vi "Acquire Image from Camera.vi"(2 "Session In":T1, 3 "AutoBalance":bool, 4 "Set":bool, 5 "Stop (F)":bool, 7 "error in":errorcluster) -> (20 "Image Out":T2(plugin-control), 22 "Buffer Number Out":u32, 26 "Stopped":bool, 27 "error out":errorcluster)   [LabVIEW 2015]
doc: "Creates, and edits acquisitions using the NI Vision Acquisition Express VI.\n\nThe NI Vision Acquisition Wizard is launched by placing the Express VI on the block diagram. Select an acquisition source and configure an acquisition using NI-IMAQ, NI-IMAQdx, or simulate an acquisition by reading an AVI or image files from a folder. After an acquisition is configured, select controls and indicators to be able to programmatically set in LabVIEW. Double-click the Vision Acquisition Express VI to edit the acquisition.\n\nNote: Any images created by the Express VI need to be disposed after use. Use the IMAQ Dispose.vi to cleanup the images output by the Express VI when they are no longer needed."
uses:
  <vilib>/userdefined/High Color/IMAQdx.ctl
  <vilib>/vision/driver/IMAQdx.llb/IMAQdx Buffer Number Mode.ctl
  <vilib>/vision/driver/IMAQdx.llb/IMAQdx Acquisition Mode.ctl
  <vilib>/vision/driver/NI_Vision_Acquisition_Software.lvlib
  <resource>/objmgr/imaqdx.rc
panel:
  out "LostBufferCount":u32
  out "error out 2":errorcluster
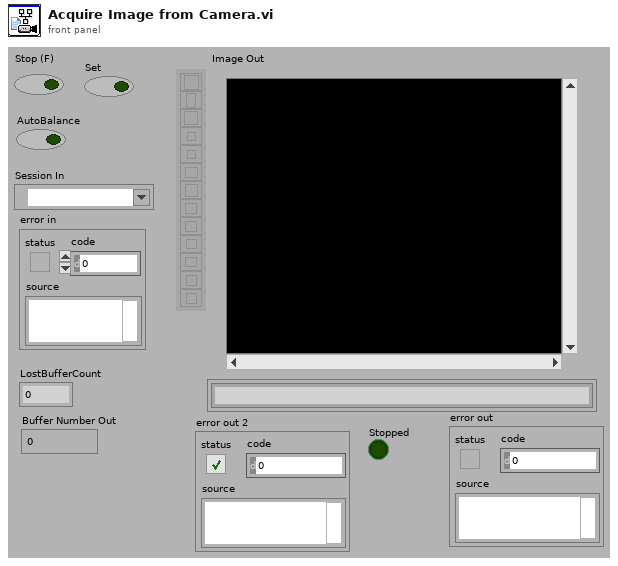
[diagram p1: front panel]
types:
  T1 = typedef "IMAQdx.ctl" = refnum<k21>
  T2 = typedef "IMAQ Image.ctl" = refnum<image>
  T3 = typedef "NI_Vision_Acquisition_Software.lvlib/IMAQdx Buffer Number Mode.ctl" = enum32{"Next", "Last", "Buffer Number", "Every", "Last New"}
  T4 = typedef "NI_Vision_Acquisition_Software.lvlib/IMAQdx Acquisition Mode.ctl" = enum32{"One Shot", "Continuous"}
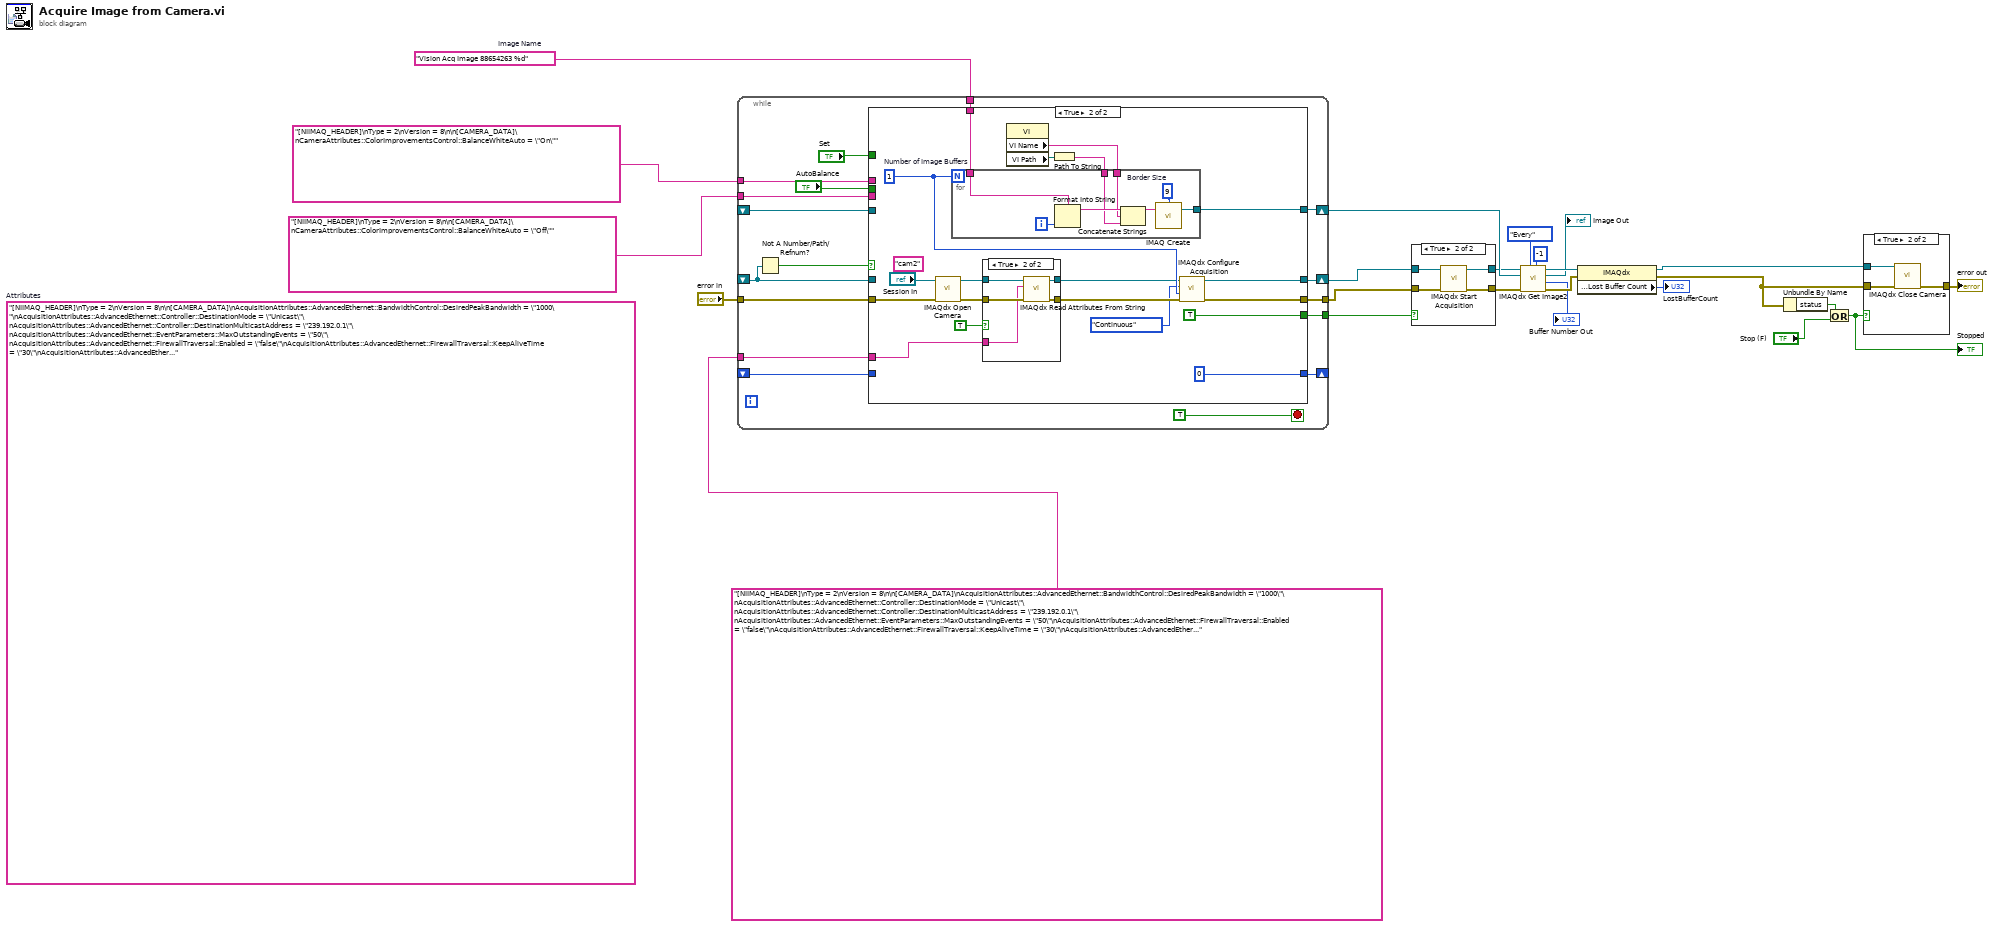
[diagram p0: block diagram]
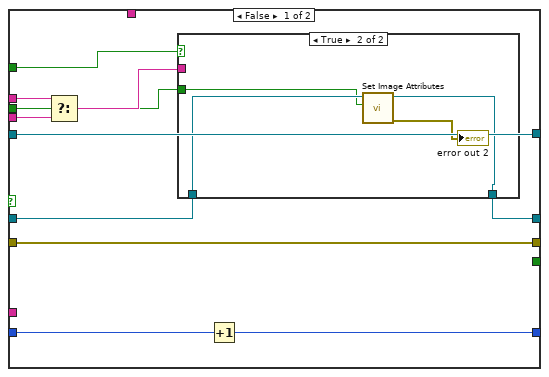
[diagram p4: hidden frame]
diagram:
  (unwired) "[NIIMAQ_HEADER]\nType = 2\nVersion = 8\n\n[CAMERA_DATA]\nAcquisitionAttributes::AdvancedEthernet::BandwidthControl::DesiredPeakBandwidth = \"1000\"\nAcquisitionAttributes::AdvancedEthernet::Controller::DestinationMode = \"Unicast\"\nAcquisitionAttributes::AdvancedEthernet::Controller::DestinationMulticastAddress = \"239.192.0.1\"\nAcquisitionAttributes::AdvancedEthernet::EventParameters::MaxOutstandingEvents = \"50\"\nAcquisitionAttributes::AdvancedEthernet::FirewallTraversal::Enabled = \"false\"\nAcquisitionAttributes::AdvancedEthernet::FirewallTraversal::KeepAliveTime = \"30\"\nAcquisitionAttributes::AdvancedEthernet::PacketReceptionParameters::KernelReceiveBufferSizeRequested = \"2000000\"\nAcquisitionAttributes::AdvancedEthernet::PacketReceptionParameters::MaximumPacketsPerReception = \"100\"\nAcquisitionAttributes::AdvancedEthernet::PacketReceptionParameters::PacketReceptionTimeout = \"450\"\nAcquisitionAttributes::AdvancedEthernet::PacketReceptionParameters::ThreadPriority = \"1\"\nAcquisitionAttributes::AdvancedEthernet::ResendParameters::MaxResendsPerPacket = \"25\"\nAcquisitionAttributes::AdvancedEthernet::ResendParameters::MemoryWindowSize = \"1024\"\nAcquisitionAttributes::AdvancedEthernet::ResendParameters::MissingPacketTimeout = \"2\"\nAcquisitionAttributes::AdvancedEthernet::ResendParameters::NewPacketTimeout = \"100\"\nAcquisitionAttributes::AdvancedEthernet::ResendParameters::ResendBatchingPercentage = \"10\"\nAcquisitionAttributes::AdvancedEthernet::ResendParameters::ResendResponseTimeout = \"2\"\nAcquisitionAttributes::AdvancedEthernet::ResendParameters::ResendsEnabled = \"true\"\nAcquisitionAttributes::AdvancedEthernet::ResendParameters::ResendThresholdPercentage = \"5\"\nAcquisitionAttributes::AdvancedEthernet::ResendParameters::ResendTimerResolution = \"1\"\nAcquisitionAttributes::AdvancedEthernet::TestPacketParameters::MaxTestPacketRetries = \"1\"\nAcquisitionAttributes::AdvancedEthernet::TestPacketParameters::TestPacketEnabled = \"true\"\nAcquisitionAttributes::AdvancedEthernet::TestPacketParameters::TestPacketTimeout = \"250\"\nAcquisitionAttributes::AdvancedGenicam::CommandTimeout = \"100\"\nAcquisitionAttributes::AdvancedGenicam::EventsEnabled = \"true\"\nAcquisitionAttributes::AdvancedGenicam::IgnoreCameraValidationErrors = \"false\"\nAcquisitionAttributes::Bayer::Algorithm = \"Bilinear\"\nAcquisitionAttributes::Bayer::GainB = \"1\"\nAcquisitionAttributes::Bayer::GainG = \"1\"\nAcquisitionAttributes::Bayer::GainR = \"1\"\nAcquisitionAttributes::Bayer::Pattern = \"Use hardware value\"\nAcquisitionAttributes::BitsPerPixel = \"Use hardware value\"\nAcquisitionAttributes::ChunkDataDecoding::ChunkDataDecodingEnabled = \"false\"\nAcquisitionAttributes::ChunkDataDecoding::MaximumChunkCopySize = \"64\"\nAcquisitionAttributes::IgnoreFirstFrame = \"false\"\nAcquisitionAttributes::ImageDecoderCopyMode = \"Auto\"\nAcquisitionAttributes::IncompleteBufferMode = \"Ignore\"\nAcquisitionAttributes::OutputImageType = \"Auto\"\nAcquisitionAttributes::OverwriteMode = \"Get Newest\"\nAcquisitionAttributes::PacketSize = \"8000\"\nAcquisitionAttributes::PixelSignedness = \"Use hardware value\"\nAcquisitionAttributes::ReceiveTimestampMode = \"None\"\nAcquisitionAttributes::ShiftPixelBits = \"false\"\nAcquisitionAttributes::SwapPixelBytes = \"false\"\nAcquisitionAttributes::Timeout = \"5000\"\nCameraAttributes::AcquisitionTrigger::AcquisitionFrameCount = \"1\"\nCameraAttributes::AcquisitionTrigger::AcquisitionFrameRateAbs = \"100\"\nCameraAttributes::AcquisitionTrigger::AcquisitionFrameRateEnable = \"true\"\nCameraAttributes::AcquisitionTrigger::ExposureAuto = \"On\"\nCameraAttributes::AcquisitionTrigger::ExposureMode = \"Timed\"\nCameraAttributes::AcquisitionTrigger::ExposureTimeRaw = \"1321\"\nCameraAttributes::AcquisitionTrigger::SensorReadoutMode = \"Normal\"\nCameraAttributes::AcquisitionTrigger::ShutterMode = \"Global\"\nCameraAttributes::AcquisitionTrigger::TriggerSelector = \"Acquisition Start\"\nCameraAttributes::AcquisitionTrigger::TriggerMode = \"Off\"\nCameraAttributes::AcquisitionTrigger::TriggerSource = \"Line 1\"\nCameraAttributes::AcquisitionTrigger::TriggerActivation = \"Rising Edge\"\nCameraAttributes::AcquisitionTrigger::TriggerDelayAbs = \"0\"\nCameraAttributes::AcquisitionTrigger::TriggerSelector = \"Frame Start\"\nCameraAttributes::AcquisitionTrigger::TriggerMode = \"Off\"\nCameraAttributes::AcquisitionTrigger::TriggerSource = \"Line 1\"\nCameraAttributes::AcquisitionTrigger::TriggerActivation = \"Rising Edge\"\nCameraAttributes::AcquisitionTrigger::TriggerDelayAbs = \"0\"\nCameraAttributes::AnalogControls::BlackLevelSelector = \"All\"\nCameraAttributes::AnalogControls::BlackLevelRaw = \"0\"\nCameraAttributes::AnalogControls::GainAuto = \"Off\"\nCameraAttributes::AnalogControls::GainSelector = \"All\"\nCameraAttributes::AnalogControls::GainRaw = \"136\"\nCameraAttributes::AnalogControls::GammaEnable = \"true\"\nCameraAttributes::AnalogControls::GammaSelector = \"SRGB\"\nCameraAttributes::AOI::CenterX = \"false\"\nCameraAttributes::AOI::CenterY = \"false\"\nCameraAttributes::AOI::Height = \"600\"\nCameraAttributes::AOI::OffsetX = \"16\"\nCameraAttributes::AOI::OffsetY = \"16\"\nCameraAttributes::AOI::Width = \"800\"\nCameraAttributes::AutoFunctions::AutoExposureTimeAbsLowerLimit = \"112\"\nCameraAttributes::AutoFunctions::AutoExposureTimeAbsUpperLimit = \"500000\"\nCameraAttributes::AutoFunctions::AutoFunctionAOIs::AutoFunctionAOISelector = \"AOI 1\"\nCameraAttributes::AutoFunctions::AutoFunctionAOIs::AutoFunctionAOIWidth = \"800\"\nCameraAttributes::AutoFunctions::AutoFunctionAOIs::AutoFunctionAOIHeight = \"600\"\nCameraAttributes::AutoFunctions::AutoFunctionAOIs::AutoFunctionAOIOffsetX = \"16\"\nCameraAttributes::AutoFunctions::AutoFunctionAOIs::AutoFunctionAOIOffsetY = \"16\"\nCameraAttributes::AutoFunctions::AutoFunctionAOIs::AutoFunctionAOISelector = \"AOI 2\"\nCameraAttributes::AutoFunctions::AutoFunctionAOIs::AutoFunctionAOIWidth = \"800\"\nCameraAttributes::AutoFunctions::AutoFunctionAOIs::AutoFunctionAOIHeight = \"600\"\nCameraAttributes::AutoFunctions::AutoFunctionAOIs::AutoFunctionAOIOffsetX = \"16\"\nCameraAttributes::AutoFunctions::AutoFunctionAOIs::AutoFunctionAOIOffsetY = \"16\"\nCameraAttributes::AutoFunctions::AutoFunctionProfile = \"Gain at minimum\"\nCameraAttributes::AutoFunctions::AutoGainRawLowerLimit = \"136\"\nCameraAttributes::AutoFunctions::AutoGainRawUpperLimit = \"542\"\nCameraAttributes::AutoFunctions::AutoTargetValue = \"128\"\nCameraAttributes::AutoFunctions::BalanceWhiteAdjustmentDampingRaw = \"1000\"\nCameraAttributes::AutoFunctions::GrayValueAdjustmentDampingRaw = \"700\"\nCameraAttributes::ChunkDataStreams::ChunkModeActive = \"false\"\nCameraAttributes::ColorImprovementsControl::BalanceRatioSelector = \"Red\"\nCameraAttributes::ColorImprovementsControl::BalanceRatioRaw = \"73\"\nCameraAttributes::ColorImprovementsControl::BalanceRatioSelector = \"Green\"\nCameraAttributes::ColorImprovementsControl::BalanceRatioRaw = \"64\"\nCameraAttributes::ColorImprovementsControl::BalanceRatioSelector = \"Blue\"\nCameraAttributes::ColorImprovementsControl::BalanceRatioRaw = \"101\"\nCameraAttributes::ColorImprovementsControl::BalanceRatioSelector = \"Red\"\nCameraAttributes::ColorImprovementsControl::BalanceWhiteAuto = \"On\"\nCameraAttributes::ColorImprovementsControl::ColorAdjustmentEnable = \"true\"\nCameraAttributes::ColorImprovementsControl::ColorAdjustmentSelector = \"Red\"\nCameraAttributes::ColorImprovementsControl::ColorAdjustmentHueRaw = \"-3\"\nCameraAttributes::ColorImprovementsControl::ColorAdjustmentSaturationRaw = \"128\"\nCameraAttributes::ColorImprovementsControl::ColorAdjustmentSelector = \"Yellow\"\nCameraAttributes::ColorImprovementsControl::ColorAdjustmentHueRaw = \"7\"\nCameraAttributes::ColorImprovementsControl::ColorAdjustmentSaturationRaw = \"124\"\nCameraAttributes::ColorImprovementsControl::ColorAdjustmentSelector = \"Green\"\nCameraAttributes::ColorImprovementsControl::ColorAdjustmentHueRaw = \"0\"\nCameraAttributes::ColorImprovementsControl::ColorAdjustmentSaturationRaw = \"138\"\nCameraAttributes::ColorImprovementsControl::ColorAdjustmentSelector = \"Cyan\"\nCameraAttributes::ColorImprovementsControl::ColorAdjustmentHueRaw = \"9\"\nCameraAttributes::ColorImprovementsControl::ColorAdjustmentSaturationRaw = \"135\"\nCameraAttributes::ColorImprovementsControl::ColorAdjustmentSelector = \"Blue\"\nCameraAttributes::ColorImprovementsControl::ColorAdjustmentHueRaw = \"-5\"\nCameraAttributes::ColorImprovementsControl::ColorAdjustmentSaturationRaw = \"126\"\nCameraAttributes::ColorImprovementsControl::ColorAdjustmentSelector = \"Magenta\"\nCameraAttributes::ColorImprovementsControl::ColorAdjustmentHueRaw = \"25\"\nCameraAttributes::ColorImprovementsControl::ColorAdjustmentSaturationRaw = \"134\"\nCameraAttributes::ColorImprovementsControl::ColorAdjustmentSelector = \"Red\"\nCameraAttributes::ColorImprovementsControl::ColorTransformationMatrixFactorRaw = \"65536\"\nCameraAttributes::ColorImprovementsControl::ColorTransformationSelector = \"RGB to RGB\"\nCameraAttributes::ColorImprovementsControl::LightSourceSelector = \"Daylight 5000 Kelvin\"\nCameraAttributes::DigitalIO::LineSelector = \"Line 1\"\nCameraAttributes::DigitalIO::LineMode = \"Input\"\nCameraAttributes::DigitalIO::LineDebouncerTimeRaw = \"10000\"\nCameraAttributes::DigitalIO::LineInverter = \"false\"\nCameraAttributes::DigitalIO::LineFormat = \"Opto-coupled\"\nCameraAttributes::DigitalIO::LineSelector = \"Line 2\"\nCameraAttributes::DigitalIO::LineMode = \"Output\"\nCameraAttributes::DigitalIO::LineInverter = \"false\"\nCameraAttributes::DigitalIO::LineSource = \"User Output 1\"\nCameraAttributes::DigitalIO::LineFormat = \"Opto-coupled\"\nCameraAttributes::DigitalIO::MinOutPulseWidthRaw = \"0\"\nCameraAttributes::DigitalIO::LineSelector = \"Line 3\"\nCameraAttributes::DigitalIO::LineMode = \"Input\"\nCameraAttributes::DigitalIO::LineDebouncerTimeRaw = \"0\"\nCameraAttributes::DigitalIO::LineInverter = \"false\"\nCameraAttributes::DigitalIO::LineFormat = \"TTL\"\nCameraAttributes::DigitalIO::LineSelector = \"Line 1\"\nCameraAttributes::DigitalIO::SyncUserOutputValueAll = \"0\"\nCameraAttributes::DigitalIO::UserOutputValueAll = \"0\"\nCameraAttributes::EventsGeneration::EventSelector = \"Exposure End\"\nCameraAttributes::EventsGeneration::EventNotification = \"Notification Off\"\nCameraAttributes::EventsGeneration::EventSelector = \"Frame Start Overtrigger\"\nCameraAttributes::EventsGeneration::EventNotification = \"Notification Off\"\nCameraAttributes::EventsGeneration::EventSelector = \"Acquisition Start Overtrigger\"\nCameraAttributes::EventsGeneration::EventNotification = \"Notification Off\"\nCameraAttributes::EventsGeneration::EventSelector = \"Frame Start\"\nCameraAttributes::EventsGeneration::EventNotification = \"Notification Off\"\nCameraAttributes::EventsGeneration::EventSelector = \"Acquisition Start\"\nCameraAttributes::EventsGeneration::EventNotification = \"Notification Off\"\nCameraAttributes::EventsGeneration::EventSelector = \"Critical Temperature\"\nCameraAttributes::EventsGeneration::EventNotification = \"Notification Off\"\nCameraAttributes::EventsGeneration::EventSelector = \"Over Temperature\"\nCameraAttributes::EventsGeneration::EventNotification = \"Notification Off\"\nCameraAttributes::EventsGeneration::EventSelector = \"Action Late\"\nCameraAttributes::EventsGeneration::EventNotification = \"Notification Off\"\nCameraAttributes::EventsGeneration::EventSelector = \"Frame Start Wait\"\nCameraAttributes::EventsGeneration::EventNotification = \"Notification Off\"\nCameraAttributes::EventsGeneration::EventSelector = \"Acquisition Start Wait\"\nCameraAttributes::EventsGeneration::EventNotification = \"Notification Off\"\nCameraAttributes::EventsGeneration::EventSelector = \"Event Overrun\"\nCameraAttributes::EventsGeneration::EventNotification = \"Notification Off\"\nCameraAttributes::EventsGeneration::EventSelector = \"Exposure End\"\nCameraAttributes::ExpertFeatureAccess::ExpertFeatureAccessSelector = \"Expert Feature 1\"\nCameraAttributes::ExpertFeatureAccess::ExpertFeatureAccessSelector = \"Expert Feature 2\"\nCameraAttributes::ExpertFeatureAccess::ExpertFeatureAccessSelector = \"Expert Feature 3\"\nCameraAttributes::ExpertFeatureAccess::ExpertFeatureAccessSelector = \"Expert Feature 4\"\nCameraAttributes::ExpertFeatureAccess::ExpertFeatureAccessSelector = \"Expert Feature 5\"\nCameraAttributes::ExpertFeatureAccess::ExpertFeatureAccessSelector = \"Expert Feature 6\"\nCameraAttributes::ExpertFeatureAccess::ExpertFeatureAccessSelector = \"Expert Feature 7\"\nCameraAttributes::ExpertFeatureAccess::ExpertFeatureAccessSelector = \"Expert Feature 8\"\nCameraAttributes::ExpertFeatureAccess::ExpertFeatureAccessSelector = \"Expert Feature 9\"\nCameraAttributes::ExpertFeatureAccess::ExpertFeatureAccessSelector = \"Expert Feature 1\"\nCameraAttributes::ImageFormat::PixelFormat = \"Bayer BG 8\"\nCameraAttributes::ImageFormat::ReverseX = \"false\"\nCameraAttributes::ImageFormat::ReverseY = \"false\"\nCameraAttributes::ImageFormat::TestImageSelector = \"Test Image Off\"\nCameraAttributes::LUTControls::LUTSelector = \"Luminance LUT\"\nCameraAttributes::LUTControls::LUTEnable = \"false\"\nCameraAttributes::LUTControls::LUTValueAll = \"000000000000000000000002000000000000000400000000000000060000000000000008000000000000000A000000000000000C000000000000000E00000000000000100000000000000012000000000000001400000000000000160000000000000018000000000000001A000000000000001C000000000000001E00000000000000200000000000000022000000000000002400000000000000260000000000000028000000000000002A000000000000002C000000000000002E00000000000000300000000000000032000000000000003400000000000000360000000000000038000000000000003A000000000000003C000000000000003E00000000000000400000000000000042000000000000004400000000000000460000000000000048000000000000004A000000000000004C000000000000004E00000000000000500000000000000052000000000000005400000000000000560000000000000058000000000000005A000000000000005C000000000000005E00000000000000600000000000000062000000000000006400000000000000660000000000000068000000000000006A000000000000006C000000000000006E00000000000000700000000000000072000000000000007400000000000000760000000000000078000000000000007A000000000000007C000000000000007E00000000000000800000000000000082000000000000008400000000000000860000000000000088000000000000008A000000000000008C000000000000008E00000000000000900000000000000092000000000000009400000000000000960000000000000098000000000000009A000000000000009C000000000000009E00000000000000A000000000000000A200000000000000A400000000000000A600000000000000A800000000000000AA00000000000000AC00000000000000AE00000000000000B000000000000000B200000000000000B400000000000000B600000000000000B800000000000000BA00000000000000BC00000000000000BE00000000000000C000000000000000C200000000000000C400000000000000C600000000000000C800000000000000CA00000000000000CC00000000000000CE00000000000000D000000000000000D200000000000000D400000000000000D600000000000000D800000000000000DA00000000000000DC00000000000000DE00000000000000E000000000000000E200000000000000E400000000000000E600000000000000E800000000000000EA00000000000000EC00000000000000EE00000000000000F000000000000000F200000000000000F400000000000000F600000000000000F800000000000000FA00000000000000FC00000000000000FE00000000000001000000000000000102000000000000010400000000000001060000000000000108000000000000010A000000000000010C000000000000010E00000000000001100000000000000112000000000000011400000000000001160000000000000118000000000000011A000000000000011C000000000000011E00000000000001200000000000000122000000000000012400000000000001260000000000000128000000000000012A000000000000012C000000000000012E00000000000001300000000000000132000000000000013400000000000001360000000000000138000000000000013A000000000000013C000000000000013E00000000000001400000000000000142000000000000014400000000000001460000000000000148000000000000014A000000000000014C000000000000014E00000000000001500000000000000152000000000000015400000000000001560000000000000158000000000000015A000000000000015C000000000000015E00000000000001600000000000000162000000000000016400000000000001660000000000000168000000000000016A000000000000016C000000000000016E00000000000001700000000000000172000000000000017400000000000001760000000000000178000000000000017A000000000000017C000000000000017E00000000000001800000000000000182000000000000018400000000000001860000000000000188000000000000018A000000000000018C000000000000018E00000000000001900000000000000192000000000000019400000000000001960000000000000198000000000000019A000000000000019C000000000000019E00000000000001A000000000000001A200000000000001A400000000000001A600000000000001A800000000000001AA00000000000001AC00000000000001AE00000000000001B000000000000001B200000000000001B400000000000001B600000000000001B800000000000001BA00000000000001BC00000000000001BE00000000000001C000000000000001C200000000000001C400000000000001C600000000000001C800000000000001CA00000000000001CC00000000000001CE00000000000001D000000000000001D200000000000001D400000000000001D600000000000001D800000000000001DA00000000000001DC00000000000001DE00000000000001E000000000000001E200000000000001E400000000000001E600000000000001E800000000000001EA00000000000001EC00000000000001EE00000000000001F000000000000001F200000000000001F400000000000001F600000000000001F800000000000001FA00000000000001FC00000000000001FE00000000000002000000000000000202000000000000020400000000000002060000000000000208000000000000020A000000000000020C000000000000020E00000000000002100000000000000212000000000000021400000000000002160000000000000218000000000000021A000000000000021C000000000000021E00000000000002200000000000000222000000000000022400000000000002260000000000000228000000000000022A000000000000022C000000000000022E00000000000002300000000000000232000000000000023400000000000002360000000000000238000000000000023A000000000000023C000000000000023E00000000000002400000000000000242000000000000024400000000000002460000000000000248000000000000024A000000000000024C000000000000024E00000000000002500000000000000252000000000000025400000000000002560000000000000258000000000000025A000000000000025C000000000000025E00000000000002600000000000000262000000000000026400000000000002660000000000000268000000000000026A000000000000026C000000000000026E00000000000002700000000000000272000000000000027400000000000002760000000000000278000000000000027A000000000000027C000000000000027E00000000000002800000000000000282000000000000028400000000000002860000000000000288000000000000028A000000000000028C000000000000028E00000000000002900000000000000292000000000000029400000000000002960000000000000298000000000000029A000000000000029C000000000000029E00000000000002A000000000000002A200000000000002A400000000000002A600000000000002A800000000000002AA00000000000002AC00000000000002AE00000000000002B000000000000002B200000000000002B400000000000002B600000000000002B800000000000002BA00000000000002BC00000000000002BE00000000000002C000000000000002C200000000000002C400000000000002C600000000000002C800000000000002CA00000000000002CC00000000000002CE00000000000002D000000000000002D200000000000002D400000000000002D600000000000002D800000000000002DA00000000000002DC00000000000002DE00000000000002E000000000000002E200000000000002E400000000000002E600000000000002E800000000000002EA00000000000002EC00000000000002EE00000000000002F000000000000002F200000000000002F400000000000002F600000000000002F800000000000002FA00000000000002FC00000000000002FE00000000000003000000000000000302000000000000030400000000000003060000000000000308000000000000030A000000000000030C000000000000030E00000000000003100000000000000312000000000000031400000000000003160000000000000318000000000000031A000000000000031C000000000000031E00000000000003200000000000000322000000000000032400000000000003260000000000000328000000000000032A000000000000032C000000000000032E00000000000003300000000000000332000000000000033400000000000003360000000000000338000000000000033A000000000000033C000000000000033E00000000000003400000000000000342000000000000034400000000000003460000000000000348000000000000034A000000000000034C000000000000034E00000000000003500000000000000352000000000000035400000000000003560000000000000358000000000000035A000000000000035C000000000000035E00000000000003600000000000000362000000000000036400000000000003660000000000000368000000000000036A000000000000036C000000000000036E00000000000003700000000000000372000000000000037400000000000003760000000000000378000000000000037A000000000000037C000000000000037E00000000000003800000000000000382000000000000038400000000000003860000000000000388000000000000038A000000000000038C000000000000038E00000000000003900000000000000392000000000000039400000000000003960000000000000398000000000000039A000000000000039C000000000000039E00000000000003A000000000000003A200000000000003A400000000000003A600000000000003A800000000000003AA00000000000003AC00000000000003AE00000000000003B000000000000003B200000000000003B400000000000003B600000000000003B800000000000003BA00000000000003BC00000000000003BE00000000000003C000000000000003C200000000000003C400000000000003C600000000000003C800000000000003CA00000000000003CC00000000000003CE00000000000003D000000000000003D200000000000003D400000000000003D600000000000003D800000000000003DA00000000000003DC00000000000003DE00000000000003E000000000000003E200000000000003E400000000000003E600000000000003E800000000000003EA00000000000003EC00000000000003EE00000000000003F000000000000003F200000000000003F400000000000003F600000000000003F800000000000003FA00000000000003FC00000000000003FE00000000\"\nCameraAttributes::RemoveParamLimits::ParameterSelector = \"Gain\"\nCameraAttributes::RemoveParamLimits::RemoveLimits = \"false\"\nCameraAttributes::RemoveParamLimits::ParameterSelector = \"Exposure Time\"\nCameraAttributes::RemoveParamLimits::RemoveLimits = \"false\"\nCameraAttributes::RemoveParamLimits::ParameterSelector = \"Target Gray Value\"\nCameraAttributes::RemoveParamLimits::RemoveLimits = \"false\"\nCameraAttributes::RemoveParamLimits::ParameterSelector = \"Gain\"\nCameraAttributes::TimerControls::CounterSelector = \"Counter 1\"\nCameraAttributes::TimerControls::CounterEventSource = \"Frame Trigger\"\nCameraAttributes::TimerControls::CounterResetSource = \"Off\"\nCameraAttributes::TimerControls::CounterSelector = \"Counter 2\"\nCameraAttributes::TimerControls::CounterEventSource = \"Frame Start\"\nCameraAttributes::TimerControls::CounterResetSource = \"Off\"\nCameraAttributes::TimerControls::TimerDelayTimebaseAbs = \"1\"\nCameraAttributes::TimerControls::TimerDurationTimebaseAbs = \"1\"\nCameraAttributes::TimerControls::TimerSelector = \"Timer 1\"\nCameraAttributes::TimerControls::TimerDurationAbs = \"4095\"\nCameraAttributes::TimerControls::TimerDurationRaw = \"4095\"\nCameraAttributes::TimerControls::TimerDelayAbs = \"0\"\nCameraAttributes::TimerControls::TimerDelayRaw = \"0\"\nCameraAttributes::TransportLayer::GevStreamChannelSelector = \"Stream Channel 0\"\nCameraAttributes::TransportLayer::GevSCFTD = \"0\"\nCameraAttributes::TransportLayer::GevSCBWR = \"10\"\nCameraAttributes::TransportLayer::GevSCBWRA = \"10\"\nCameraAttributes::UserDefinedValues::UserDefinedValueSelector = \"Value 1\"\nCameraAttributes::UserDefinedValues::UserDefinedValue = \"0\"\nCameraAttributes::UserDefinedValues::UserDefinedValueSelector = \"Value 2\"\nCameraAttributes::UserDefinedValues::UserDefinedValue = \"0\"\nCameraAttributes::UserDefinedValues::UserDefinedValueSelector = \"Value 3\"\nCameraAttributes::UserDefinedValues::UserDefinedValue = \"0\"\nCameraAttributes::UserDefinedValues::UserDefinedValueSelector = \"Value 4\"\nCameraAttributes::UserDefinedValues::UserDefinedValue = \"0\"\nCameraAttributes::UserDefinedValues::UserDefinedValueSelector = \"Value 5\"\nCameraAttributes::UserDefinedValues::UserDefinedValue = \"0\"\nCameraAttributes::UserDefinedValues::UserDefinedValueSelector = \"Value 1\"\n"  # Attributes
  w6 = "Vision Acq Image 88654263 %d"  # Image Name
  n1 = while {
    shift-right: [w41] -> w17
    shift-left: _ -> [w33]
    tunnel: [w40] -> w23
    tunnel: "error in" -> [w39]
    shift-right: [w37] -> w19
    shift-left: _ -> [w36]
    shift-right: [w35] -> _
    shift-left: _ -> [w34]
    tunnel: [w32] -> w14
    tunnel: w6 -> [w31]
    tunnel: "[NIIMAQ_HEADER]\nType = 2\nVersion = 8\n\n[CAMERA_DATA]\nAcquisitionAttributes::AdvancedEthernet::BandwidthControl::DesiredPeakBandwidth = \"1000\"\nAcquisitionAttributes::AdvancedEthernet::Controller::DestinationMode = \"Unicast\"\nAcquisitionAttributes::AdvancedEthernet::Controller::DestinationMulticastAddress = \"239.192.0.1\"\nAcquisitionAttributes::AdvancedEthernet::EventParameters::MaxOutstandingEvents = \"50\"\nAcquisitionAttributes::AdvancedEthernet::FirewallTraversal::Enabled = \"false\"\nAcquisitionAttributes::AdvancedEthernet::FirewallTraversal::KeepAliveTime = \"30\"\nAcquisitionAttributes::AdvancedEthernet::PacketReceptionParameters::KernelReceiveBufferSizeRequested = \"2000000\"\nAcquisitionAttributes::AdvancedEthernet::PacketReceptionParameters::MaximumPacketsPerReception = \"100\"\nAcquisitionAttributes::AdvancedEthernet::PacketReceptionParameters::PacketReceptionTimeout = \"450\"\nAcquisitionAttributes::AdvancedEthernet::PacketReceptionParameters::ThreadPriority = \"1\"\nAcquisitionAttributes::AdvancedEthernet::ResendParameters::MaxResendsPerPacket = \"25\"\nAcquisitionAttributes::AdvancedEthernet::ResendParameters::MemoryWindowSize = \"1024\"\nAcquisitionAttributes::AdvancedEthernet::ResendParameters::MissingPacketTimeout = \"2\"\nAcquisitionAttributes::AdvancedEthernet::ResendParameters::NewPacketTimeout = \"100\"\nAcquisitionAttributes::AdvancedEthernet::ResendParameters::ResendBatchingPercentage = \"10\"\nAcquisitionAttributes::AdvancedEthernet::ResendParameters::ResendResponseTimeout = \"2\"\nAcquisitionAttributes::AdvancedEthernet::ResendParameters::ResendsEnabled = \"true\"\nAcquisitionAttributes::AdvancedEthernet::ResendParameters::ResendThresholdPercentage = \"5\"\nAcquisitionAttributes::AdvancedEthernet::ResendParameters::ResendTimerResolution = \"1\"\nAcquisitionAttributes::AdvancedEthernet::TestPacketParameters::MaxTestPacketRetries = \"1\"\nAcquisitionAttributes::AdvancedEthernet::TestPacketParameters::TestPacketEnabled = \"true\"\nAcquisitionAttributes::AdvancedEthernet::TestPacketParameters::TestPacketTimeout = \"250\"\nAcquisitionAttributes::AdvancedGenicam::CommandTimeout = \"100\"\nAcquisitionAttributes::AdvancedGenicam::EventsEnabled = \"true\"\nAcquisitionAttributes::AdvancedGenicam::IgnoreCameraValidationErrors = \"false\"\nAcquisitionAttributes::Bayer::Algorithm = \"Bilinear\"\nAcquisitionAttributes::Bayer::GainB = \"0.877538834319664396\"\nAcquisitionAttributes::Bayer::GainG = \"0.864790174043026272\"\nAcquisitionAttributes::Bayer::GainR = \"0.854384386209105284\"\nAcquisitionAttributes::Bayer::Pattern = \"Use hardware value\"\nAcquisitionAttributes::BitsPerPixel = \"Use hardware value\"\nAcquisitionAttributes::ChunkDataDecoding::ChunkDataDecodingEnabled = \"false\"\nAcquisitionAttributes::ChunkDataDecoding::MaximumChunkCopySize = \"64\"\nAcquisitionAttributes::IgnoreFirstFrame = \"false\"\nAcquisitionAttributes::ImageDecoderCopyMode = \"Auto\"\nAcquisitionAttributes::IncompleteBufferMode = \"Ignore\"\nAcquisitionAttributes::OutputImageType = \"Auto\"\nAcquisitionAttributes::OverwriteMode = \"Get Newest\"\nAcquisitionAttributes::PacketSize = \"8000\"\nAcquisitionAttributes::PixelSignedness = \"Use hardware value\"\nAcquisitionAttributes::ReceiveTimestampMode = \"None\"\nAcquisitionAttributes::ShiftPixelBits = \"false\"\nAcquisitionAttributes::SwapPixelBytes = \"false\"\nAcquisitionAttributes::Timeout = \"5000\"\nCameraAttributes::AcquisitionTrigger::AcquisitionFrameCount = \"1\"\nCameraAttributes::AcquisitionTrigger::AcquisitionFrameRateAbs = \"100\"\nCameraAttributes::AcquisitionTrigger::AcquisitionFrameRateEnable = \"true\"\nCameraAttributes::AcquisitionTrigger::ExposureAuto = \"Off\"\nCameraAttributes::AcquisitionTrigger::ExposureMode = \"Timed\"\nCameraAttributes::AcquisitionTrigger::ExposureTimeRaw = \"2500\"\nCameraAttributes::AcquisitionTrigger::SensorReadoutMode = \"Normal\"\nCameraAttributes::AcquisitionTrigger::ShutterMode = \"Global\"\nCameraAttributes::AcquisitionTrigger::TriggerSelector = \"Acquisition Start\"\nCameraAttributes::AcquisitionTrigger::TriggerMode = \"Off\"\nCameraAttributes::AcquisitionTrigger::TriggerSource = \"Line 1\"\nCameraAttributes::AcquisitionTrigger::TriggerActivation = \"Rising Edge\"\nCameraAttributes::AcquisitionTrigger::TriggerDelayAbs = \"0\"\nCameraAttributes::AcquisitionTrigger::TriggerSelector = \"Frame Start\"\nCameraAttributes::AcquisitionTrigger::TriggerMode = \"Off\"\nCameraAttributes::AcquisitionTrigger::TriggerSource = \"Line 1\"\nCameraAttributes::AcquisitionTrigger::TriggerActivation = \"Rising Edge\"\nCameraAttributes::AcquisitionTrigger::TriggerDelayAbs = \"0\"\nCameraAttributes::AnalogControls::BlackLevelSelector = \"All\"\nCameraAttributes::AnalogControls::BlackLevelRaw = \"0\"\nCameraAttributes::AnalogControls::GainAuto = \"Off\"\nCameraAttributes::AnalogControls::GainSelector = \"All\"\nCameraAttributes::AnalogControls::GainRaw = \"136\"\nCameraAttributes::AnalogControls::GammaEnable = \"true\"\nCameraAttributes::AnalogControls::GammaSelector = \"SRGB\"\nCameraAttributes::AOI::CenterX = \"false\"\nCameraAttributes::AOI::CenterY = \"false\"\nCameraAttributes::AOI::Height = \"600\"\nCameraAttributes::AOI::OffsetX = \"0\"\nCameraAttributes::AOI::OffsetY = \"0\"\nCameraAttributes::AOI::Width = \"800\"\nCameraAttributes::AutoFunctions::AutoExposureTimeAbsLowerLimit = \"112\"\nCameraAttributes::AutoFunctions::AutoExposureTimeAbsUpperLimit = \"500000\"\nCameraAttributes::AutoFunctions::AutoFunctionAOIs::AutoFunctionAOISelector = \"AOI 1\"\nCameraAttributes::AutoFunctions::AutoFunctionAOIs::AutoFunctionAOIWidth = \"800\"\nCameraAttributes::AutoFunctions::AutoFunctionAOIs::AutoFunctionAOIHeight = \"600\"\nCameraAttributes::AutoFunctions::AutoFunctionAOIs::AutoFunctionAOIOffsetX = \"16\"\nCameraAttributes::AutoFunctions::AutoFunctionAOIs::AutoFunctionAOIOffsetY = \"16\"\nCameraAttributes::AutoFunctions::AutoFunctionAOIs::AutoFunctionAOISelector = \"AOI 2\"\nCameraAttributes::AutoFunctions::AutoFunctionAOIs::AutoFunctionAOIWidth = \"800\"\nCameraAttributes::AutoFunctions::AutoFunctionAOIs::AutoFunctionAOIHeight = \"600\"\nCameraAttributes::AutoFunctions::AutoFunctionAOIs::AutoFunctionAOIOffsetX = \"16\"\nCameraAttributes::AutoFunctions::AutoFunctionAOIs::AutoFunctionAOIOffsetY = \"16\"\nCameraAttributes::AutoFunctions::AutoFunctionProfile = \"Gain at minimum\"\nCameraAttributes::AutoFunctions::AutoGainRawLowerLimit = \"136\"\nCameraAttributes::AutoFunctions::AutoGainRawUpperLimit = \"542\"\nCameraAttributes::AutoFunctions::AutoTargetValue = \"128\"\nCameraAttributes::AutoFunctions::BalanceWhiteAdjustmentDampingRaw = \"1000\"\nCameraAttributes::AutoFunctions::GrayValueAdjustmentDampingRaw = \"700\"\nCameraAttributes::ChunkDataStreams::ChunkModeActive = \"false\"\nCameraAttributes::ColorImprovementsControl::BalanceRatioSelector = \"Red\"\nCameraAttributes::ColorImprovementsControl::BalanceRatioRaw = \"158\"\nCameraAttributes::ColorImprovementsControl::BalanceRatioSelector = \"Green\"\nCameraAttributes::ColorImprovementsControl::BalanceRatioRaw = \"117\"\nCameraAttributes::ColorImprovementsControl::BalanceRatioSelector = \"Blue\"\nCameraAttributes::ColorImprovementsControl::BalanceRatioRaw = \"64\"\nCameraAttributes::ColorImprovementsControl::BalanceRatioSelector = \"Red\"\nCameraAttributes::ColorImprovementsControl::BalanceWhiteAuto = \"Off\"\nCameraAttributes::ColorImprovementsControl::ColorAdjustmentEnable = \"true\"\nCameraAttributes::ColorImprovementsControl::ColorAdjustmentSelector = \"Red\"\nCameraAttributes::ColorImprovementsControl::ColorAdjustmentHueRaw = \"-3\"\nCameraAttributes::ColorImprovementsControl::ColorAdjustmentSaturationRaw = \"128\"\nCameraAttributes::ColorImprovementsControl::ColorAdjustmentSelector = \"Yellow\"\nCameraAttributes::ColorImprovementsControl::ColorAdjustmentHueRaw = \"7\"\nCameraAttributes::ColorImprovementsControl::ColorAdjustmentSaturationRaw = \"124\"\nCameraAttributes::ColorImprovementsControl::ColorAdjustmentSelector = \"Green\"\nCameraAttributes::ColorImprovementsControl::ColorAdjustmentHueRaw = \"0\"\nCameraAttributes::ColorImprovementsControl::ColorAdjustmentSaturationRaw = \"138\"\nCameraAttributes::ColorImprovementsControl::ColorAdjustmentSelector = \"Cyan\"\nCameraAttributes::ColorImprovementsControl::ColorAdjustmentHueRaw = \"9\"\nCameraAttributes::ColorImprovementsControl::ColorAdjustmentSaturationRaw = \"135\"\nCameraAttributes::ColorImprovementsControl::ColorAdjustmentSelector = \"Blue\"\nCameraAttributes::ColorImprovementsControl::ColorAdjustmentHueRaw = \"-5\"\nCameraAttributes::ColorImprovementsControl::ColorAdjustmentSaturationRaw = \"126\"\nCameraAttributes::ColorImprovementsControl::ColorAdjustmentSelector = \"Magenta\"\nCameraAttributes::ColorImprovementsControl::ColorAdjustmentHueRaw = \"25\"\nCameraAttributes::ColorImprovementsControl::ColorAdjustmentSaturationRaw = \"134\"\nCameraAttributes::ColorImprovementsControl::ColorAdjustmentSelector = \"Red\"\nCameraAttributes::ColorImprovementsControl::ColorTransformationMatrixFactorRaw = \"65536\"\nCameraAttributes::ColorImprovementsControl::ColorTransformationSelector = \"RGB to RGB\"\nCameraAttributes::ColorImprovementsControl::LightSourceSelector = \"Daylight 5000 Kelvin\"\nCameraAttributes::DigitalIO::LineSelector = \"Line 1\"\nCameraAttributes::DigitalIO::LineMode = \"Input\"\nCameraAttributes::DigitalIO::LineDebouncerTimeRaw = \"10000\"\nCameraAttributes::DigitalIO::LineInverter = \"false\"\nCameraAttributes::DigitalIO::LineFormat = \"Opto-coupled\"\nCameraAttributes::DigitalIO::LineSelector = \"Line 2\"\nCameraAttributes::DigitalIO::LineMode = \"Output\"\nCameraAttributes::DigitalIO::LineInverter = \"false\"\nCameraAttributes::DigitalIO::LineSource = \"User Output 1\"\nCameraAttributes::DigitalIO::LineFormat = \"Opto-coupled\"\nCameraAttributes::DigitalIO::MinOutPulseWidthRaw = \"0\"\nCameraAttributes::DigitalIO::LineSelector = \"Line 3\"\nCameraAttributes::DigitalIO::LineMode = \"Input\"\nCameraAttributes::DigitalIO::LineDebouncerTimeRaw = \"0\"\nCameraAttributes::DigitalIO::LineInverter = \"false\"\nCameraAttributes::DigitalIO::LineFormat = \"TTL\"\nCameraAttributes::DigitalIO::LineSelector = \"Line 1\"\nCameraAttributes::DigitalIO::SyncUserOutputValueAll = \"0\"\nCameraAttributes::DigitalIO::UserOutputValueAll = \"0\"\nCameraAttributes::EventsGeneration::EventSelector = \"Exposure End\"\nCameraAttributes::EventsGeneration::EventNotification = \"Notification Off\"\nCameraAttributes::EventsGeneration::EventSelector = \"Frame Start Overtrigger\"\nCameraAttributes::EventsGeneration::EventNotification = \"Notification Off\"\nCameraAttributes::EventsGeneration::EventSelector = \"Acquisition Start Overtrigger\"\nCameraAttributes::EventsGeneration::EventNotification = \"Notification Off\"\nCameraAttributes::EventsGeneration::EventSelector = \"Frame Start\"\nCameraAttributes::EventsGeneration::EventNotification = \"Notification Off\"\nCameraAttributes::EventsGeneration::EventSelector = \"Acquisition Start\"\nCameraAttributes::EventsGeneration::EventNotification = \"Notification Off\"\nCameraAttributes::EventsGeneration::EventSelector = \"Critical Temperature\"\nCameraAttributes::EventsGeneration::EventNotification = \"Notification Off\"\nCameraAttributes::EventsGeneration::EventSelector = \"Over Temperature\"\nCameraAttributes::EventsGeneration::EventNotification = \"Notification Off\"\nCameraAttributes::EventsGeneration::EventSelector = \"Action Late\"\nCameraAttributes::EventsGeneration::EventNotification = \"Notification Off\"\nCameraAttributes::EventsGeneration::EventSelector = \"Frame Start Wait\"\nCameraAttributes::EventsGeneration::EventNotification = \"Notification Off\"\nCameraAttributes::EventsGeneration::EventSelector = \"Acquisition Start Wait\"\nCameraAttributes::EventsGeneration::EventNotification = \"Notification Off\"\nCameraAttributes::EventsGeneration::EventSelector = \"Event Overrun\"\nCameraAttributes::EventsGeneration::EventNotification = \"Notification Off\"\nCameraAttributes::EventsGeneration::EventSelector = \"Exposure End\"\nCameraAttributes::ExpertFeatureAccess::ExpertFeatureAccessSelector = \"Expert Feature 1\"\nCameraAttributes::ExpertFeatureAccess::ExpertFeatureAccessSelector = \"Expert Feature 2\"\nCameraAttributes::ExpertFeatureAccess::ExpertFeatureAccessSelector = \"Expert Feature 3\"\nCameraAttributes::ExpertFeatureAccess::ExpertFeatureAccessSelector = \"Expert Feature 4\"\nCameraAttributes::ExpertFeatureAccess::ExpertFeatureAccessSelector = \"Expert Feature 5\"\nCameraAttributes::ExpertFeatureAccess::ExpertFeatureAccessSelector = \"Expert Feature 6\"\nCameraAttributes::ExpertFeatureAccess::ExpertFeatureAccessSelector = \"Expert Feature 7\"\nCameraAttributes::ExpertFeatureAccess::ExpertFeatureAccessSelector = \"Expert Feature 8\"\nCameraAttributes::ExpertFeatureAccess::ExpertFeatureAccessSelector = \"Expert Feature 9\"\nCameraAttributes::ExpertFeatureAccess::ExpertFeatureAccessSelector = \"Expert Feature 1\"\nCameraAttributes::ImageFormat::PixelFormat = \"Bayer BG 8\"\nCameraAttributes::ImageFormat::ReverseX = \"false\"\nCameraAttributes::ImageFormat::ReverseY = \"false\"\nCameraAttributes::ImageFormat::TestImageSelector = \"Test Image Off\"\nCameraAttributes::LUTControls::LUTSelector = \"Luminance LUT\"\nCameraAttributes::LUTControls::LUTEnable = \"false\"\nCameraAttributes::LUTControls::LUTValueAll = \"000000000000000000000002000000000000000400000000000000060000000000000008000000000000000A000000000000000C000000000000000E00000000000000100000000000000012000000000000001400000000000000160000000000000018000000000000001A000000000000001C000000000000001E00000000000000200000000000000022000000000000002400000000000000260000000000000028000000000000002A000000000000002C000000000000002E00000000000000300000000000000032000000000000003400000000000000360000000000000038000000000000003A000000000000003C000000000000003E00000000000000400000000000000042000000000000004400000000000000460000000000000048000000000000004A000000000000004C000000000000004E00000000000000500000000000000052000000000000005400000000000000560000000000000058000000000000005A000000000000005C000000000000005E00000000000000600000000000000062000000000000006400000000000000660000000000000068000000000000006A000000000000006C000000000000006E00000000000000700000000000000072000000000000007400000000000000760000000000000078000000000000007A000000000000007C000000000000007E00000000000000800000000000000082000000000000008400000000000000860000000000000088000000000000008A000000000000008C000000000000008E00000000000000900000000000000092000000000000009400000000000000960000000000000098000000000000009A000000000000009C000000000000009E00000000000000A000000000000000A200000000000000A400000000000000A600000000000000A800000000000000AA00000000000000AC00000000000000AE00000000000000B000000000000000B200000000000000B400000000000000B600000000000000B800000000000000BA00000000000000BC00000000000000BE00000000000000C000000000000000C200000000000000C400000000000000C600000000000000C800000000000000CA00000000000000CC00000000000000CE00000000000000D000000000000000D200000000000000D400000000000000D600000000000000D800000000000000DA00000000000000DC00000000000000DE00000000000000E000000000000000E200000000000000E400000000000000E600000000000000E800000000000000EA00000000000000EC00000000000000EE00000000000000F000000000000000F200000000000000F400000000000000F600000000000000F800000000000000FA00000000000000FC00000000000000FE00000000000001000000000000000102000000000000010400000000000001060000000000000108000000000000010A000000000000010C000000000000010E00000000000001100000000000000112000000000000011400000000000001160000000000000118000000000000011A000000000000011C000000000000011E00000000000001200000000000000122000000000000012400000000000001260000000000000128000000000000012A000000000000012C000000000000012E00000000000001300000000000000132000000000000013400000000000001360000000000000138000000000000013A000000000000013C000000000000013E00000000000001400000000000000142000000000000014400000000000001460000000000000148000000000000014A000000000000014C000000000000014E00000000000001500000000000000152000000000000015400000000000001560000000000000158000000000000015A000000000000015C000000000000015E00000000000001600000000000000162000000000000016400000000000001660000000000000168000000000000016A000000000000016C000000000000016E00000000000001700000000000000172000000000000017400000000000001760000000000000178000000000000017A000000000000017C000000000000017E00000000000001800000000000000182000000000000018400000000000001860000000000000188000000000000018A000000000000018C000000000000018E00000000000001900000000000000192000000000000019400000000000001960000000000000198000000000000019A000000000000019C000000000000019E00000000000001A000000000000001A200000000000001A400000000000001A600000000000001A800000000000001AA00000000000001AC00000000000001AE00000000000001B000000000000001B200000000000001B400000000000001B600000000000001B800000000000001BA00000000000001BC00000000000001BE00000000000001C000000000000001C200000000000001C400000000000001C600000000000001C800000000000001CA00000000000001CC00000000000001CE00000000000001D000000000000001D200000000000001D400000000000001D600000000000001D800000000000001DA00000000000001DC00000000000001DE00000000000001E000000000000001E200000000000001E400000000000001E600000000000001E800000000000001EA00000000000001EC00000000000001EE00000000000001F000000000000001F200000000000001F400000000000001F600000000000001F800000000000001FA00000000000001FC00000000000001FE00000000000002000000000000000202000000000000020400000000000002060000000000000208000000000000020A000000000000020C000000000000020E00000000000002100000000000000212000000000000021400000000000002160000000000000218000000000000021A000000000000021C000000000000021E00000000000002200000000000000222000000000000022400000000000002260000000000000228000000000000022A000000000000022C000000000000022E00000000000002300000000000000232000000000000023400000000000002360000000000000238000000000000023A000000000000023C000000000000023E00000000000002400000000000000242000000000000024400000000000002460000000000000248000000000000024A000000000000024C000000000000024E00000000000002500000000000000252000000000000025400000000000002560000000000000258000000000000025A000000000000025C000000000000025E00000000000002600000000000000262000000000000026400000000000002660000000000000268000000000000026A000000000000026C000000000000026E00000000000002700000000000000272000000000000027400000000000002760000000000000278000000000000027A000000000000027C000000000000027E00000000000002800000000000000282000000000000028400000000000002860000000000000288000000000000028A000000000000028C000000000000028E00000000000002900000000000000292000000000000029400000000000002960000000000000298000000000000029A000000000000029C000000000000029E00000000000002A000000000000002A200000000000002A400000000000002A600000000000002A800000000000002AA00000000000002AC00000000000002AE00000000000002B000000000000002B200000000000002B400000000000002B600000000000002B800000000000002BA00000000000002BC00000000000002BE00000000000002C000000000000002C200000000000002C400000000000002C600000000000002C800000000000002CA00000000000002CC00000000000002CE00000000000002D000000000000002D200000000000002D400000000000002D600000000000002D800000000000002DA00000000000002DC00000000000002DE00000000000002E000000000000002E200000000000002E400000000000002E600000000000002E800000000000002EA00000000000002EC00000000000002EE00000000000002F000000000000002F200000000000002F400000000000002F600000000000002F800000000000002FA00000000000002FC00000000000002FE00000000000003000000000000000302000000000000030400000000000003060000000000000308000000000000030A000000000000030C000000000000030E00000000000003100000000000000312000000000000031400000000000003160000000000000318000000000000031A000000000000031C000000000000031E00000000000003200000000000000322000000000000032400000000000003260000000000000328000000000000032A000000000000032C000000000000032E00000000000003300000000000000332000000000000033400000000000003360000000000000338000000000000033A000000000000033C000000000000033E00000000000003400000000000000342000000000000034400000000000003460000000000000348000000000000034A000000000000034C000000000000034E00000000000003500000000000000352000000000000035400000000000003560000000000000358000000000000035A000000000000035C000000000000035E00000000000003600000000000000362000000000000036400000000000003660000000000000368000000000000036A000000000000036C000000000000036E00000000000003700000000000000372000000000000037400000000000003760000000000000378000000000000037A000000000000037C000000000000037E00000000000003800000000000000382000000000000038400000000000003860000000000000388000000000000038A000000000000038C000000000000038E00000000000003900000000000000392000000000000039400000000000003960000000000000398000000000000039A000000000000039C000000000000039E00000000000003A000000000000003A200000000000003A400000000000003A600000000000003A800000000000003AA00000000000003AC00000000000003AE00000000000003B000000000000003B200000000000003B400000000000003B600000000000003B800000000000003BA00000000000003BC00000000000003BE00000000000003C000000000000003C200000000000003C400000000000003C600000000000003C800000000000003CA00000000000003CC00000000000003CE00000000000003D000000000000003D200000000000003D400000000000003D600000000000003D800000000000003DA00000000000003DC00000000000003DE00000000000003E000000000000003E200000000000003E400000000000003E600000000000003E800000000000003EA00000000000003EC00000000000003EE00000000000003F000000000000003F200000000000003F400000000000003F600000000000003F800000000000003FA00000000000003FC00000000000003FE00000000\"\nCameraAttributes::RemoveParamLimits::ParameterSelector = \"Gain\"\nCameraAttributes::RemoveParamLimits::RemoveLimits = \"false\"\nCameraAttributes::RemoveParamLimits::ParameterSelector = \"Exposure Time\"\nCameraAttributes::RemoveParamLimits::RemoveLimits = \"false\"\nCameraAttributes::RemoveParamLimits::ParameterSelector = \"Target Gray Value\"\nCameraAttributes::RemoveParamLimits::RemoveLimits = \"false\"\nCameraAttributes::RemoveParamLimits::ParameterSelector = \"Gain\"\nCameraAttributes::TimerControls::CounterSelector = \"Counter 1\"\nCameraAttributes::TimerControls::CounterEventSource = \"Frame Trigger\"\nCameraAttributes::TimerControls::CounterResetSource = \"Off\"\nCameraAttributes::TimerControls::CounterSelector = \"Counter 2\"\nCameraAttributes::TimerControls::CounterEventSource = \"Frame Start\"\nCameraAttributes::TimerControls::CounterResetSource = \"Off\"\nCameraAttributes::TimerControls::TimerDelayTimebaseAbs = \"1\"\nCameraAttributes::TimerControls::TimerDurationTimebaseAbs = \"1\"\nCameraAttributes::TimerControls::TimerSelector = \"Timer 1\"\nCameraAttributes::TimerControls::TimerDurationAbs = \"4095\"\nCameraAttributes::TimerControls::TimerDurationRaw = \"4095\"\nCameraAttributes::TimerControls::TimerDelayAbs = \"0\"\nCameraAttributes::TimerControls::TimerDelayRaw = \"0\"\nCameraAttributes::TransportLayer::GevStreamChannelSelector = \"Stream Channel 0\"\nCameraAttributes::TransportLayer::GevSCFTD = \"0\"\nCameraAttributes::TransportLayer::GevSCBWR = \"10\"\nCameraAttributes::TransportLayer::GevSCBWRA = \"10\"\nCameraAttributes::UserDefinedValues::UserDefinedValueSelector = \"Value 1\"\nCameraAttributes::UserDefinedValues::UserDefinedValue = \"0\"\nCameraAttributes::UserDefinedValues::UserDefinedValueSelector = \"Value 2\"\nCameraAttributes::UserDefinedValues::UserDefinedValue = \"0\"\nCameraAttributes::UserDefinedValues::UserDefinedValueSelector = \"Value 3\"\nCameraAttributes::UserDefinedValues::UserDefinedValue = \"0\"\nCameraAttributes::UserDefinedValues::UserDefinedValueSelector = \"Value 4\"\nCameraAttributes::UserDefinedValues::UserDefinedValue = \"0\"\nCameraAttributes::UserDefinedValues::UserDefinedValueSelector = \"Value 5\"\nCameraAttributes::UserDefinedValues::UserDefinedValue = \"0\"\nCameraAttributes::UserDefinedValues::UserDefinedValueSelector = \"Value 1\"\n" -> [w30]
    tunnel: "[NIIMAQ_HEADER]\nType = 2\nVersion = 8\n\n[CAMERA_DATA]\nCameraAttributes::ColorImprovementsControl::BalanceWhiteAuto = \"On\"" -> [w26]
    tunnel: "[NIIMAQ_HEADER]\nType = 2\nVersion = 8\n\n[CAMERA_DATA]\nCameraAttributes::ColorImprovementsControl::BalanceWhiteAuto = \"Off\"" -> [w25]
    stop <- TRUE stop-if-true
    n2 = Not A Number/Path/Refnum?(number/path/refnum=w33) -> (NaN/Path/Refnum?=w29:bool)
    n3 = case shown="True" w29 {
      tunnel: [w46 w75] -> w41
      tunnel: w33 -> [w47 _]
      tunnel: [w52 w74] -> w40
      tunnel: w39 -> [w52 w76]
      tunnel: [w51 w73] -> w37
      tunnel: w36 -> [w51 _]
      tunnel: [w49 0] -> w35
      tunnel: w34 -> [w50 _]
      tunnel: [_ TRUE] -> w32
      tunnel: w31 -> [_ w60]
      tunnel: w30 -> [_ w59]
      tunnel: "Set" -> [w48 _]
      tunnel: "AutoBalance" -> [w42 _]
      tunnel: w26 -> [w45 _]
      tunnel: w25 -> [w44 _]
      frame False {
        n4 = Select(t=w45, s=w42, f=w44) -> (s? t:f=w43:string)
        n5 = case shown="True" w48 {
          tunnel: w47 -> [w53 w57]
          tunnel: [w53 w56] -> w46
          tunnel: w43 -> [_ _]
          tunnel: w42 -> [_ w55]
          frame False {
          }
          frame True {
            n6 = call "Set Image Attributes.vi"("AutoBalance"=w55, "Refnum in"=w57) -> ("error out"=→"error out 2":errorcluster, "Refnum out"=w56:T1)  [unwired: 8 in]
          }
        }
        n7 = Increment(x=w50) -> (x+1=w49:i32)
      }
      frame True {
        w72 = u32 1  # Number of Image Buffers
        (unwired) "cam2" ("Interface Name")
        n8 = call <vilib>:"IMAQdx Open Camera.vi"("error in"=w76, "Session In"="Session In") -> ("error out"=w66:errorcluster, "Session Out"=w67:T1)  [unwired: 1 in, 7 out]
        n9 = case shown="True" TRUE ("Init Attributes") {
          tunnel: w67 -> [w78 w83]
          tunnel: w66 -> [w77 w82]
          tunnel: [w78 w81] -> w65
          tunnel: [w77 w80] -> w64
          tunnel: w59 -> [_ w79]
          frame False {
          }
          frame True {
            n10 = call <vilib>:"IMAQdx Read Attributes From String.vi"("error in"=w82, "Attributes String In"=w79, "Session In"=w83) -> ("error out"=w80:errorcluster, "Session Out"=w81:T1)  [unwired: 7 out]
          }
        }
        n11 = property class="VI"() -> ("VI Name"=w69:string, "VI Path"=w70:path)  [unwired: 2 in, 2 out]
        n12 = Path To String(path=w70) -> (string=w68:string)
        n13 = for "For Loop_template0" {
          N: w72 -> [_]
          tunnel: [w91] -> w73
          tunnel: w69 -> [w87]
          tunnel: w68 -> [w86]
          tunnel: w60 -> [w85]
          i -> [w90]
          w84 = 9  # Border Size
          n14 = Format Into String(format string=w85, w90) -> (resulting string=w89:string)  [unwired: 2 in, 1 out]
          n15 = Concatenate Strings(w89, w87, w86) -> (w88:string)
          n16 = call "IMAQ Create"("Border Size"=w84, "Image Name"=w88) -> ("New Image"=w91:T2)  [unwired: 2 in, 2 out]
        }
        n17 = call <vilib>:"IMAQdx Configure Acquisition.vi"("error in"=w64, "Number of Buffers"=w72, "Continuous?"=IMAQdx_Acquisition_Mode."Continuous", "Session In"=w65) -> ("error out"=w74:errorcluster, "Session Out"=w75:T1)  [unwired: 6 out]
      }
    }
  }
  n18 = case shown="True" w14 {
    tunnel: w17 -> [w93 w97]
    tunnel: w23 -> [w92 w96]
    tunnel: [w92 w95] -> w15
    tunnel: [w93 w94] -> w16
    frame False {
    }
    frame True {
      n19 = call <vilib>:"IMAQdx Start Acquisition.vi"("error in"=w96, "Session In"=w97) -> ("error out"=w95:errorcluster, "Session Out"=w94:T1)  [unwired: 8 out]
    }
  }
  n20 = call <vilib>:"IMAQdx Get Image2.vi"("Timeout (ms)"=-1, "Buffer Number Mode (Next)"=IMAQdx_Buffer_Number_Mode."Every", "error in"=w15, "Image In"=w19, "Session In"=w16) -> ("error out"=w21:errorcluster, "Buffer Number Out"=→"Buffer Number Out":u32, "Image Out"=→"Image Out":T2, "Session Out"=w22:T1)  [unwired: 3 in]
  n21 = property class="IMAQdx"(reference=w22, error in=w21) -> (reference out=w11:T1, error out=w18:errorcluster, "Status Information:Lost Buffer Count"=→"LostBufferCount":u32)
  n22 = Unbundle By Name(w18) -> ("status"=w7:bool)
  n23 = Or(x=w7, y="Stop (F)") -> (x .or. y?=w8:bool)
  "Stopped" <- w8
  n24 = case "Case Structure_template1" shown="True" w8 {
    tunnel: [w98 w100] -> w10
    tunnel: w18 -> [w98 w101]
    tunnel: w11 -> [_ w99]
    frame False {
    }
    frame True {
      n25 = call <vilib>:"IMAQdx Close Camera.vi"("error in"=w101, "Session In"=w99) -> ("error out"=w100:errorcluster)  [unwired: 9 out]
    }
  }
  "error out" <- w10
